vi "Configure Basic Dual Channel FFT.vi"(0 "VISA resource name":refnum<visa-resource-name>, 1 "Start Frequency (0 mHz)":dbl, 2 "Stop Frequency (0 mHz)":dbl, 3 "DC Correction Mode (0: dcmNone)":i32(ring) items=["dcmNone", "dcmMean", "dcmPkPK"], 5 "Analyzer (0: A0)":i32(ring) items=["A0", "A1"], 7 "Lines (0: fftl32k)":i32(ring) items=["fftl32k", "fftl16k", "fftl8k", "fftl4k", "fftl2k", "fftl1k", "fftl512", "fftl256"], 9 "Span (0: fftFsDiv2)":i32(ring) items=["fftFsDiv2", "fftFsDiv4", "fftFsDiv8", "fftFsDiv16", "fftFsDiv32", "fftFsDiv64", "fftFsDiv128", "fftFsDiv256", "fftFsDiv512", "fftFsDiv1024"], 11 "error in (no error)":errorcluster, 12 "Center Frequency (0 mHz)":dbl, 13 "FFT Window (0: fftBlackmanHarris)":i32(ring) items=["fftBlackmanHarris", "fftHann", "fftHamming", "fftEquiripple", "fftFlattop", "fftGaussian", "fftKaiser", "fftUniform", "fftRifeVincent4", "fftRifeVincent5", "fftRifeVincent10", "fftBlackmanHarris7", "fftVariable"]) -> (4 "VISA resource name out":refnum<visa-resource-name>, 15 "error out":errorcluster)   [LabVIEW 2014, in "Stanford Research SR1.lvlib"]
doc: "Configures the attributes for the Basic Dual Channel FFT."
uses:
  Stanford Research SR1.lvlib
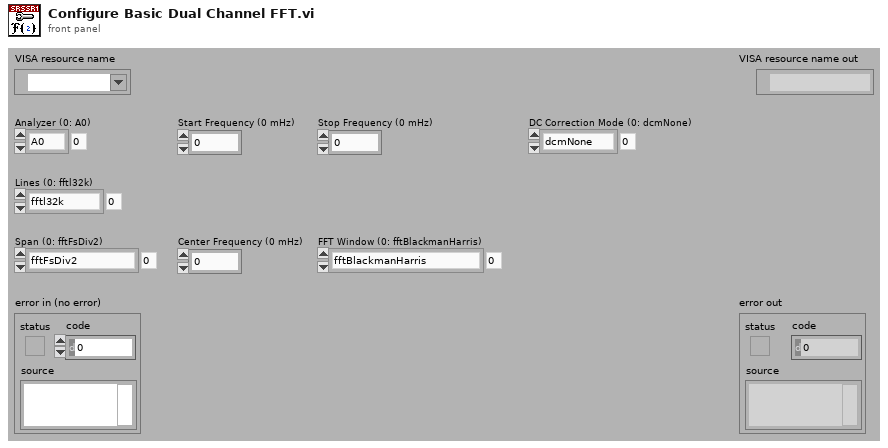
[diagram p1: front panel]
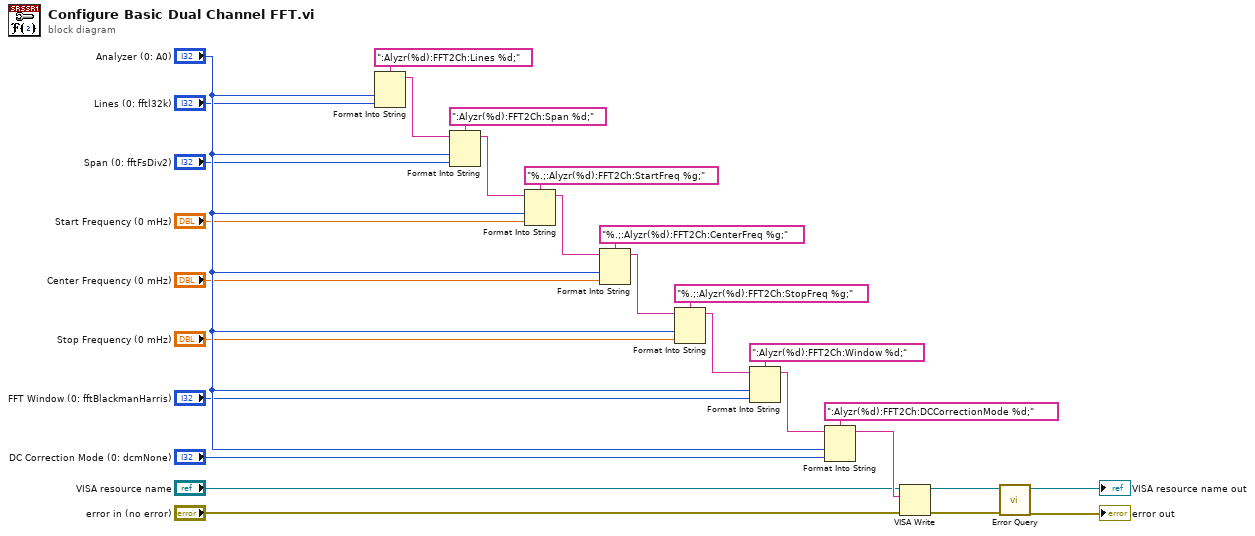
[diagram p0: block diagram]
diagram:
  n1 = Format Into String(format string=":Alyzr(%d):FFT2Ch:Lines %d;", "Analyzer (0: A0)", "Lines (0: fftl32k)") -> (resulting string=w27:string)  [unwired: 2 in, 1 out]
  n2 = Format Into String(format string=":Alyzr(%d):FFT2Ch:Span %d;", initial string=w27, "Analyzer (0: A0)", "Span (0: fftFsDiv2)") -> (resulting string=w25:string)  [unwired: 1 in, 1 out]
  n3 = Format Into String(format string="%.;:Alyzr(%d):FFT2Ch:StartFreq %g;", initial string=w25, "Analyzer (0: A0)", "Start Frequency (0 mHz)") -> (resulting string=w23:string)  [unwired: 1 in, 1 out]
  n4 = Format Into String(format string="%.;:Alyzr(%d):FFT2Ch:CenterFreq %g;", initial string=w23, "Analyzer (0: A0)", "Center Frequency (0 mHz)") -> (resulting string=w21:string)  [unwired: 1 in, 1 out]
  n5 = Format Into String(format string="%.;:Alyzr(%d):FFT2Ch:StopFreq %g;", initial string=w21, "Analyzer (0: A0)", "Stop Frequency (0 mHz)") -> (resulting string=w19:string)  [unwired: 1 in, 1 out]
  n6 = Format Into String(format string=":Alyzr(%d):FFT2Ch:Window %d;", initial string=w19, "Analyzer (0: A0)", "FFT Window (0: fftBlackmanHarris)") -> (resulting string=w17:string)  [unwired: 1 in, 1 out]
  n7 = Format Into String(format string=":Alyzr(%d):FFT2Ch:DCCorrectionMode %d;", initial string=w17, "Analyzer (0: A0)", "DC Correction Mode (0: dcmNone)") -> (resulting string=w15:string)  [unwired: 1 in, 1 out]
  n8 = VISA Write(VISA resource name="VISA resource name", write buffer=w15, error in (no error)="error in (no error)") -> (VISA resource name out=w12:refnum<visa-resource-name>, error out=w11:errorcluster)  [unwired: 1 out]
  n9 = call "Error Query.vi"("error in (no error)"=w11, "VISA resource name"=w12) -> ("error out"=→"error out":errorcluster, "VISA resource name out"=→"VISA resource name out":refnum<visa-resource-name>)  [unwired: 6 in, 2 out]
